vi "SoftLimitBlockers.vi"(11 "Motor Ref":T1) -> ()   [LabVIEW 2015]
uses:
  Framework/Detailed Motor Type Def.ctl
  <vilib>/Rock Robotics/WPI/MotorControl/WPI_MotorControlDeviceRef.ctl
  <vilib>/Rock Robotics/WPI/MotorControl/WPI_MotorControlType.ctl
  <vilib>/Rock Robotics/SystemInterfaces/DIO/FPGA_DIOPWMChannel.ctl
  <vilib>/Rock Robotics/WPI/PWM/WPI_PWMDeadband.ctl
  <vilib>/Rock Robotics/WPI/CAN/Jaguar/SubVIs/WPI_CANJaguar_ControlMode.ctl
  <vilib>/Rock Robotics/WPI/CAN/TalonSRX/WPI_CANTalonSRX_APIControlMode.ctl
  Framework/Robot Global Data.vi
  Shooter Global.vi
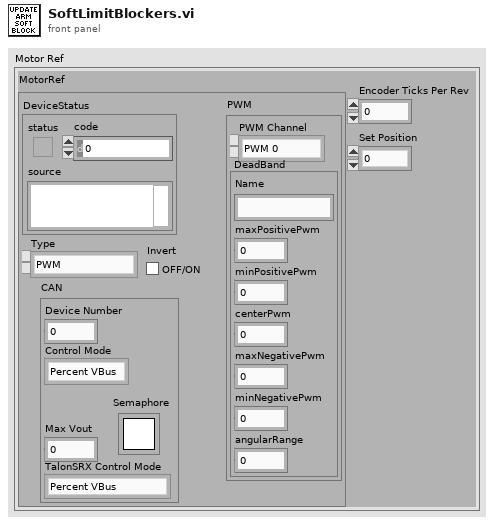
[diagram p1: front panel]
types:
  T1 = typedef "Detailed Motor Type Def.ctl" = cluster{"MotorRef":T2, "Encoder Ticks Per Rev":dbl, "Set Position":dbl}
  T2 = typedef "WPI_MotorControlDeviceRef.ctl" = cluster{"DeviceStatus":errorcluster, "Type":T3, "PWM":cluster{"PWM Channel":T4, "DeadBand":T5}, "CAN":cluster{"Device Number":u8, "Control Mode":T6, "Semaphore":T7, "Max Vout":dbl, "TalonSRX Control Mode":T8}, "Invert":bool}
  T3 = typedef "WPI_MotorControlType.ctl" = enum16{"PWM", "CAN", "CANTalonSRX"}
  T4 = typedef "FPGA_DIOPWMChannel.ctl" = enum8{"PWM 0", "PWM 1", "PWM 2", "PWM 3", "PWM 4", "PWM 5", "PWM 6", "PWM 7", "PWM 8", "PWM 9", "PWM MXP 0", "PWM MXP 1", "PWM MXP 2", "PWM MXP 3", "PWM MXP 4", "PWM MXP 5", "PWM MXP 6", "PWM MXP 7", "PWM MXP 8", "PWM MXP 9", "Invalid"}
  T5 = typedef "WPI_PWMDeadband.ctl" = cluster{"Name":string, "maxPositivePwm":i32, "minPositivePwm":i32, "centerPwm":i32, "maxNegativePwm":i32, "minNegativePwm":i32, "angularRange":u16}
  T6 = typedef "WPI_CANJaguar_ControlMode.ctl" = enum8{"Percent VBus", "Current", "Speed", "Position", "Voltage"}
  T7 = typedef "Semaphore RefNum" = refnum<k1>
  T8 = typedef "WPI_CANTalonSRX_APIControlMode.ctl" = enum8{"Percent VBus", "Speed", "Position", "Slave", "Unchanged / Invalid", "Voltage Compensation", "Current", "Motion Profile"}
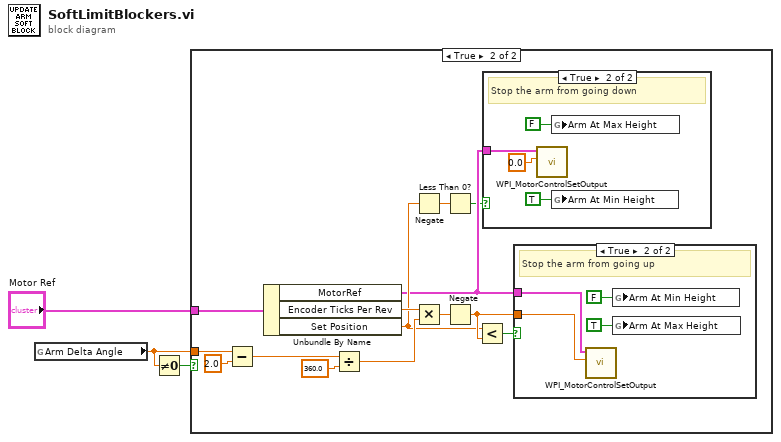
[diagram p0: block diagram]
diagram:
  n1 = global read "Robot Global Data.vi" "Arm Delta Angle"() -> (w2:dbl)
  n2 = Not Equal To 0?(x=w2) -> (x != 0?=w1:bool)
  n3 = case shown="True" w1 {
    tunnel: "Motor Ref" -> [_ w17]
    tunnel: w2 -> [_ w4]
    frame False {
    }
    frame True {
      n4 = Subtract(x=w4, y=2.0) -> (x-y=w14:dbl)
      n5 = Unbundle By Name(w17) -> ("MotorRef"=w7:T2, "Encoder Ticks Per Rev"=w12:dbl, "Set Position"=w8:dbl)
      n6 = Divide(x=w14, y=360.0) -> (x/y=w15:dbl)
      n7 = Negate(x=w8) -> (-x=w9:dbl)
      n8 = Multiply(x=w12, y=w15) -> (x*y=w10:dbl)
      n9 = Less Than 0?(x=w9) -> (x < 0?=w6:bool)
      n10 = Negate(x=w10) -> (-x=w11:dbl)
      n11 = Less?(x=w8, y=w11) -> (x < y?=w5:bool)
      n12 = case shown="True" w6 {
        tunnel: w7 -> [_ w25]
        frame False {
        }
        frame True {
          # "Stop the arm from going down"
          n13 = call <vilib>:"WPI_MotorControlSetOutput.vi"("Output"=0.0, "MotorControlDevRef"=w25) -> ()  [unwired: 7 in, 3 out]
          n14 = global write "Shooter Global.vi" "Arm At Max Height"(FALSE) -> ()
          n15 = global write "Shooter Global.vi" "Arm At Min Height"(TRUE) -> ()
        }
      }
      n16 = case shown="True" w5 {
        tunnel: w11 -> [_ w18]
        tunnel: w7 -> [_ w21]
        frame False {
        }
        frame True {
          # "Stop the arm from going up"
          n17 = call <vilib>:"WPI_MotorControlSetOutput.vi"("Output"=w18, "MotorControlDevRef"=w21) -> ()  [unwired: 7 in, 3 out]
          n18 = global write "Shooter Global.vi" "Arm At Min Height"(FALSE) -> ()
          n19 = global write "Shooter Global.vi" "Arm At Max Height"(TRUE) -> ()
        }
      }
    }
  }
